vi "Power PID View.vi"(11 "Model in":refnum<class "Model.lvclass">) -> ()   [LabVIEW 2016, in "M1M3SupportEUI_Views.lvlib"]
uses:
  M1M3SupportEUI_Views.lvlib
  Model/Model.lvclass
  SALLV_m1m3/DataTypes/PIDData.ctl
  SALLV_m1m3/DataTypes/logevent_PIDInfo.ctl
  M1M3 Support Events/M1M3 Support Events.lvclass/M1M3 Support Events.ctl
  SALLV_m1m3/DataTypes/command_UpdatePID.ctl
  SALLV_m1m3/DataTypes/command_ResetPID.ctl
  SALLV_m1m3/DataTypes/command_TurnPowerOn.ctl
  M1M3 Support Events/M1M3 Support Events.lvclass
  SALLV_m1m3/SALLV_m1m3.lvlib
  EUI Events/EUI Events.lvclass
panel:
  out "Any":bool
  out "Power Warning Time Stamp":timestamp
  out "Power Status Time Stamp":timestamp
  out "AuxComDMismatch":bool
  out "MainComDMismatch":bool
  out "AuxComCMismatch":bool
  out "MainComCMismatch":bool
  out "AuxComBMismatch":bool
  out "MainComBMismatch":bool
  out "AuxComAMismatch":bool
  out "MainComAMismatch":bool
  out "AuxOutD":bool
  out "AuxOutC":bool
  out "AuxOutB":bool
  out "AuxOutA":bool
  out "AuxComD":bool
  out "AuxComC":bool
  out "AuxComB":bool
  out "AuxComA":bool
  out "MainOutD":bool
  out "MainOutC":bool
  out "MainOutB":bool
  out "MainOutA":bool
  out "MainComD":bool
  out "MainComC":bool
  out "MainComB":bool
  out "MainComA":bool
  in  "Aux All":bool
  in  "Aux D":bool
  in  "Aux C":bool
  in  "Aux B":bool
  in  "Aux A":bool
  in  "Main All":bool
  in  "Main D":bool
  in  "Main C":bool
  in  "Main B":bool
  in  "MainA":bool
  out "PID Event Time Stamp":timestamp
  in  "logevent_PIDInfo":T1={"Timestamp"=0.0, "Timestep[6]"=[0.0, 0.0, 0.0, 0.0, 0.0, 0.0], "P[6]"=[0.0, 0.0, 0.0, 0.0, 0.0, 0.0], "I[6]"=[0.0, 0.0, 0.0, 0.0, 0.0, 0.0], "D[6]"=[0.0, 0.0, 0.0, 0.0, 0.0, 0.0], "N[6]"=[0.0, 0.0, 0.0, 0.0, 0.0, 0.0], "CalculatedA[6]"=[0.0, 0.0, 0.0, 0.0, 0.0, 0.0], "CalculatedB[6]"=[0.0, 0.0, 0.0, 0.0, 0.0, 0.0], "CalculatedC[6]"=[0.0, 0.0, 0.0, 0.0, 0.0, 0.0], "CalculatedD[6]"=[0.0, 0.0, 0.0, 0.0, 0.0, 0.0], "CalculatedE[6]"=[0.0, 0.0, 0.0, 0.0, 0.0, 0.0], "priority"=0}
  in  "PID":enum16{"0", "1", "2", "3", "4", "5"}(ring)
  in  "N":dbl
  in  "D":dbl
  in  "I":dbl
  in  "P":dbl
  in  "Timestep":dbl
  in  "PID Data/Event Type":string(combo)
  out "6":string
  out "5":string
  out "4":string
  out "3":string
  out "2":string
  out "1":string
  in  "PIDData":T2={"Timestamp"=0.0, "Setpoint[6]"=[0.0, 0.0, 0.0, 0.0, 0.0, 0.0], "Measurement[6]"=[0.0, 0.0, 0.0, 0.0, 0.0, 0.0], "Error[6]"=[0.0, 0.0, 0.0, 0.0, 0.0, 0.0], "ErrorT1[6]"=[0.0, 0.0, 0.0, 0.0, 0.0, 0.0], "ErrorT2[6]"=[0.0, 0.0, 0.0, 0.0, 0.0, 0.0], "Control[6]"=[0.0, 0.0, 0.0, 0.0, 0.0, 0.0], "ControlT1[6]"=[0.0, 0.0, 0.0, 0.0, 0.0, 0.0], "ControlT2[6]"=[0.0, 0.0, 0.0, 0.0, 0.0, 0.0]}
  in  "Reset PID Button":bool
  in  "Update PID Button":bool
  out "Controls Power Network Current":string
  out "Light Power Network Current":string
  out "Power Network D Current":string
  out "Power Network C Current":string
  out "Power Network B Current":string
  out "Power Network A Current":string
  out "PID TelemetryTime Stamp":timestamp
  out "Power Time Stamp":timestamp
  # "Power"
  # "PID"
  # "Commands"
  # "Data"
  # "Commands"
  # "Main"
  # "Aux"
  # "PID"
  # "P"
  # "A"
  # "Timestep"
  # "I"
  # "B"
  # "C"
  # "D"
  # "D"
  # "N"
  # "ALL"
  # "Data & Events"
  # "Events"
  # "Status"
  # "Main"
  # "Auxiliary"
  # "Commanded"
  # "Commanded"
  # "Output"
  # "Output"
  # "A"
  # "3"
  # "1"
  # "2"
  # "B"
  # "C"
  # "6"
  # "4"
  # "5"
  # "D"
  # "Warnings - Mismatch"
  # "A"
  # "B"
  # "C"
  # "D"
  # "Main"
  # "Any -->"
  # "Auxiliary"
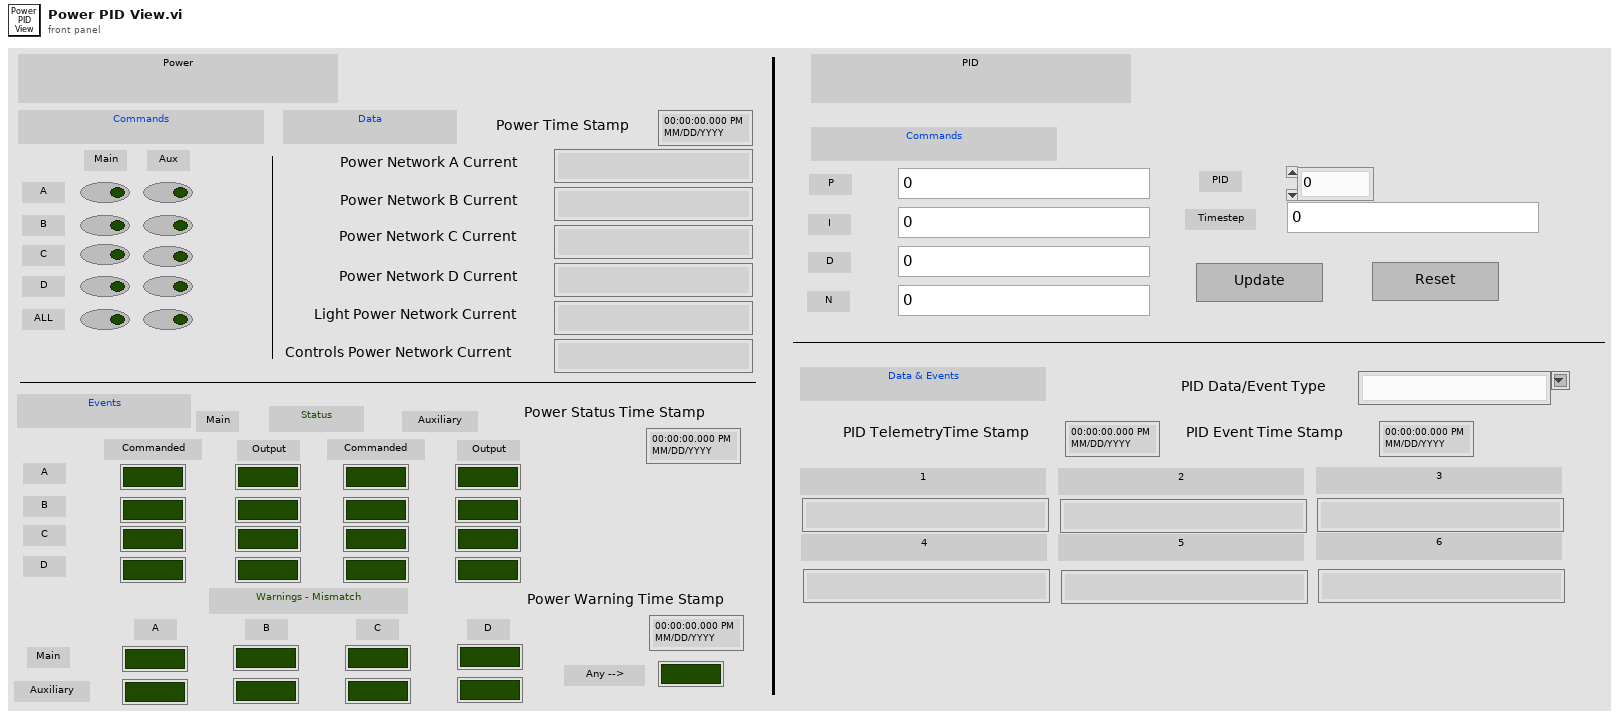
[diagram p1: front panel]
types:
  T1 = typedef "SALLV_m1m3.lvlib/logevent_PIDInfo.ctl" = cluster{"Timestamp":dbl, "Timestep[6]":dbl[], "P[6]":dbl[], "I[6]":dbl[], "D[6]":dbl[], "N[6]":dbl[], "CalculatedA[6]":dbl[], "CalculatedB[6]":dbl[], "CalculatedC[6]":dbl[], "CalculatedD[6]":dbl[], "CalculatedE[6]":dbl[], "priority":i32}
  T2 = typedef "SALLV_m1m3.lvlib/PIDData.ctl" = cluster{"Timestamp":dbl, "Setpoint[6]":dbl[], "Measurement[6]":dbl[], "Error[6]":dbl[], "ErrorT1[6]":dbl[], "ErrorT2[6]":dbl[], "Control[6]":dbl[], "ControlT1[6]":dbl[], "ControlT2[6]":dbl[]}
  T3 = typedef "M1M3SupportEUI_TypeDefs.lvlib/M1M3 Support Events.ctl" = cluster{"Inclinometer  Data":refnum<user-event>, "IMS Data":refnum<user-event>, "SAL Connected":refnum<user-event>, "Accelerometer Data":refnum<user-event>, "OuterLoop Data":refnum<user-event>, "ErrorCode Event":refnum<user-event>, "InterlockStatus Event":refnum<user-event>, "InterlockWarning Event":refnum<user-event>, "Gyro Data":refnum<user-event>, "HP Actuator Info Event":refnum<user-event>, " FA Info Event":refnum<user-event>, "HP Monitor Info Event":refnum<user-event>, "FA Data":refnum<user-event>, "HP Actuator data":refnum<user-event>, "HP Monitor data":refnum<user-event>, "Air Supply Status Event":refnum<user-event>, "Air Supply Warning Event":refnum<user-event>, "Power Data":refnum<user-event>, "PID Data":refnum<user-event>, "PID Info Event":refnum<user-event>, "Power Status Event":refnum<user-event>, "Power Supply Status Event":refnum<user-event>, "Power Warning Event":refnum<user-event>, "Summary State Event":refnum<user-event>, "Detailed State Event":refnum<user-event>, "FA Force Warning Event":refnum<user-event>, "FA Warning Event":refnum<user-event>, "FA State Event":refnum<user-event>, "Applied AberrationForces Event":refnum<user-event>, "Applied Acceleration Forcces Event":refnum<user-event>, "Applied Azimuth Forces Event":refnum<user-event>, "Applied Active Optic Forces Event":refnum<user-event>, "Applied Balance Forces Event":refnum<user-event>, "Applied Cylinder Forces Event":refnum<user-event>, "Applied Elevation Forces Event":refnum<user-event>, "Applied Forces Event":refnum<user-event>, "Applied Offset Forces Event":refnum<user-event>, "Applied Static Forces Event":refnum<user-event>, "Applied Thermal Forces Event":refnum<user-event>, "Applied Velocity Forces Event":refnum<user-event>, "Rejected Aberration Force Event":refnum<user-event>, "Rejected Acceleration Forces Event":refnum<user-event>, "Rejected Active Optic Forces Event":refnum<user-event>, "Rejected Azimuth Forces Event":refnum<user-event>, "Rejected Balance Forces Event":refnum<user-event>, "Rejected Cylinder Forces Event":refnum<user-event>, "Rejected Elevation Forces Event":refnum<user-event>, "Rejected Forces Event":refnum<user-event>, "Rejected Offset Forces Event":refnum<user-event>, "Rejected Static Forces Event":refnum<user-event>, "Rejected Thermal Forces Event":refnum<user-event>, "Rejected Velocity Forces Event":refnum<user-event>, "Command Rejection Event":refnum<user-event>, "Setting Verions Event":refnum<user-event>, "Settings Applied Event":refnum<user-event>, "HP Actuator State Event":refnum<user-event>, "HP Actuator Warning Event":refnum<user-event>, "HP Monitor State Event":refnum<user-event>, "HP Monitor Warning Event":refnum<user-event>, "Accelerometer Warning Event":refnum<user-event>, "Applied Settings Match Start Event":refnum<user-event>, "Cell Light Status Event ":refnum<user-event>, "Cell Light Warning Event":refnum<user-event>, "Displacement Sensor Warning Event":refnum<user-event>, "Force Setpoint Warning Event":refnum<user-event>, "Gyro Warning Event ":refnum<user-event>, "ILC Warning Event ":refnum<user-event>, "Inclinometer Sensor Warning Event ":refnum<user-event>}
  T4 = enum16{"", "DetailedState_DetailedStates_DisabledState", "DetailedState_DetailedStates_EnabledState", "DetailedState_DetailedStates_FaultState", "DetailedState_DetailedStates_OfflineState", "DetailedState_DetailedStates_StandbyState", "DetailedState_DetailedStates_ParkedState", "DetailedState_DetailedStates_RaisingState", "DetailedState_DetailedStates_ActiveState", "DetailedState_DetailedStates_LoweringState", "DetailedState_DetailedStates_EngineeringState", "DetailedState_DetailedStates_ParkedEngineeringState", "DetailedState_DetailedStates_RaisingEngineeringState", "DetailedState_DetailedStates_ActiveEngineeringState", "DetailedState_DetailedStates_LoweringEngineeringState", "DetailedState_DetailedStates_LoweringFaultState", "DetailedState_DetailedStates_ProfileHardpointCorrectionState"}
  T5 = typedef "SALLV_m1m3.lvlib/command_UpdatePID.ctl" = cluster{"PID":i16, "Timestep":dbl, "P":dbl, "I":dbl, "D":dbl, "N":dbl}
  T6 = typedef "SALLV_m1m3.lvlib/command_ResetPID.ctl" = cluster{"PID":i16}
  T7 = typedef "SALLV_m1m3.lvlib/command_TurnPowerOn.ctl" = cluster{"TurnPowerNetworkAOn":bool, "TurnPowerNetworkBOn":bool, "TurnPowerNetworkCOn":bool, "TurnPowerNetworkDOn":bool, "TurnAuxPowerNetworkAOn":bool, "TurnAuxPowerNetworkBOn":bool, "TurnAuxPowerNetworkCOn":bool, "TurnAuxPowerNetworkDOn":bool}
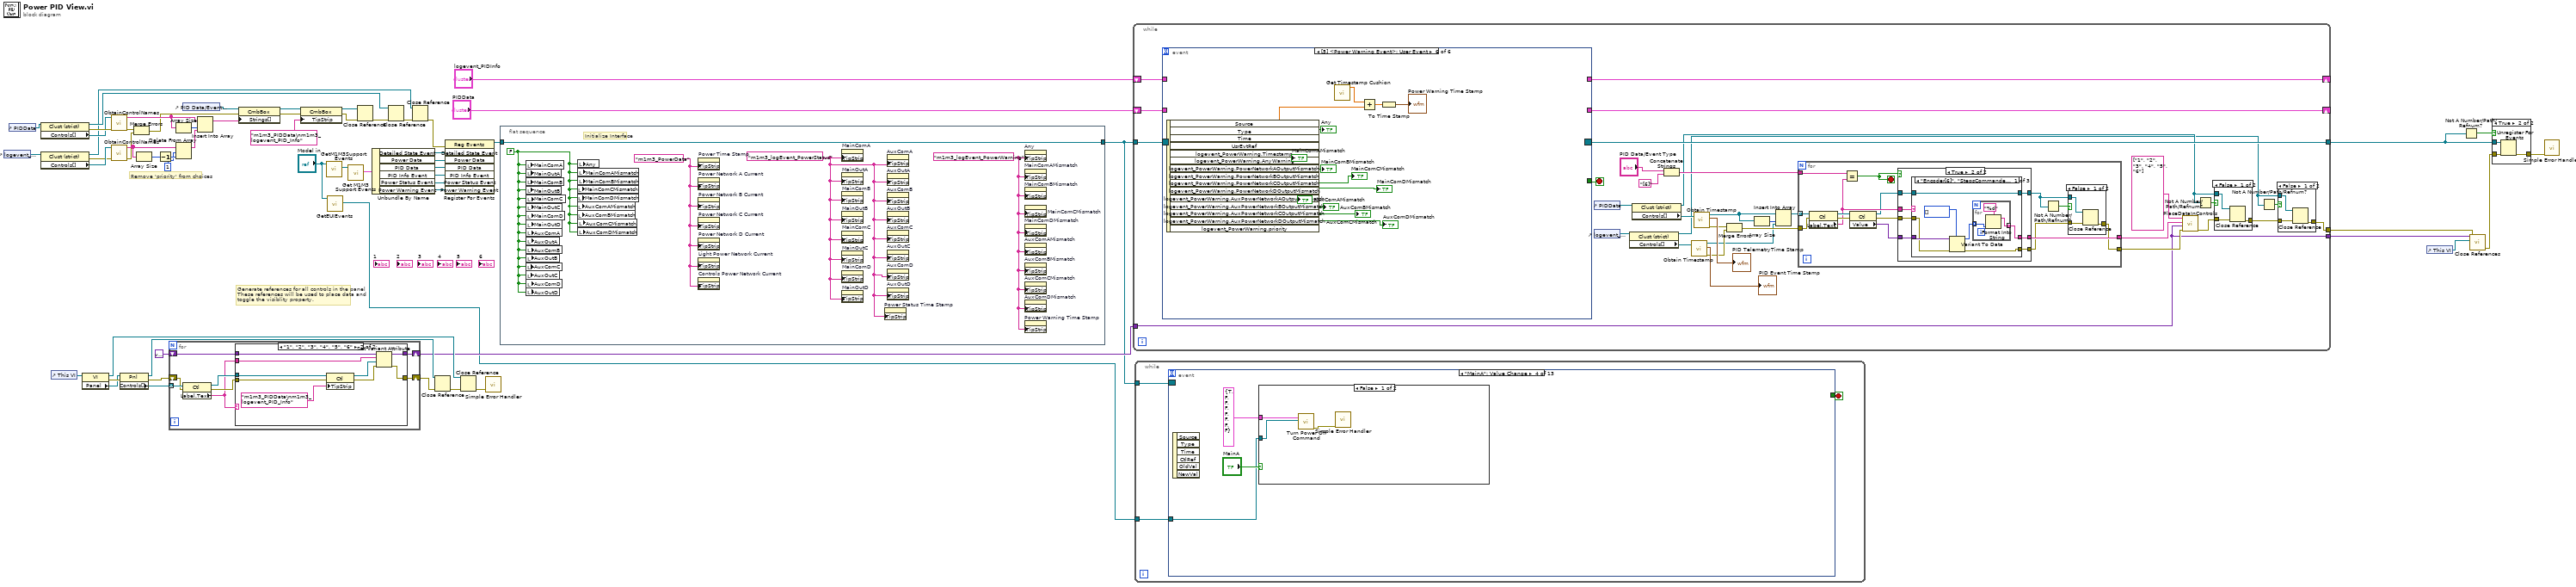
[diagram p0: block diagram]
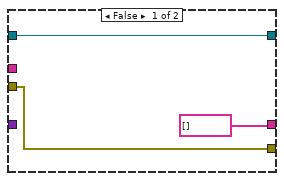
[diagram p4: hidden frame]
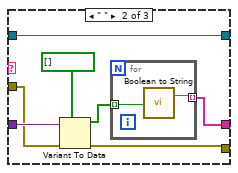
[diagram p5: hidden frame]
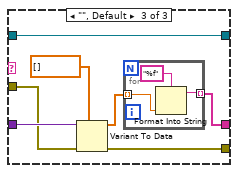
[diagram p6: hidden frame]
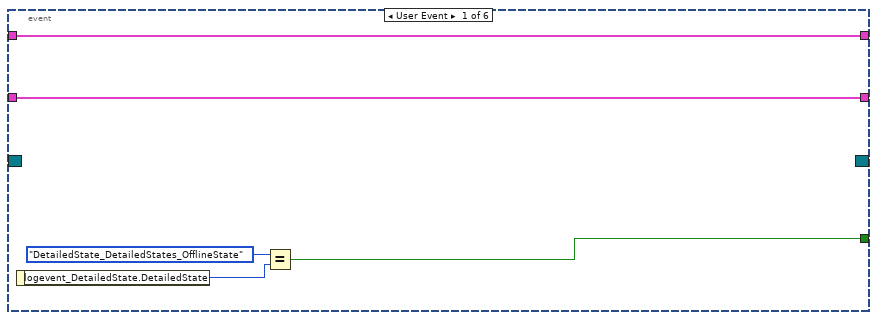
[diagram p7: hidden frame]
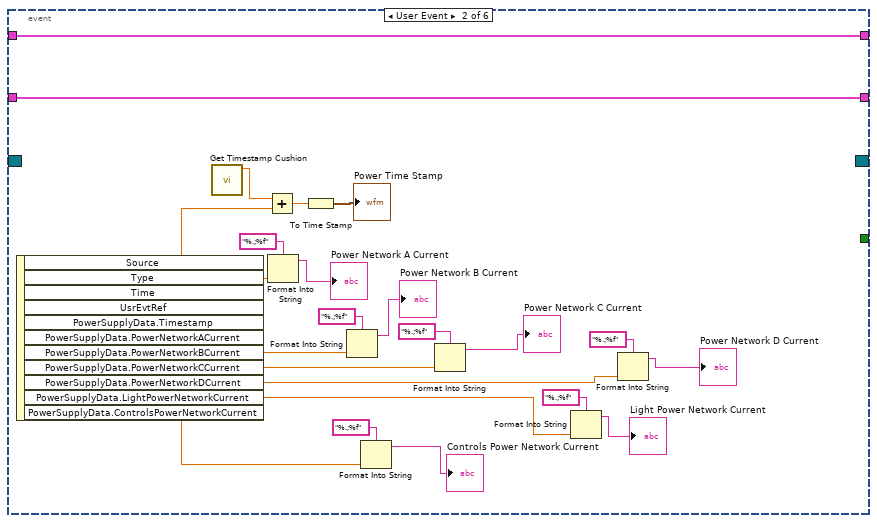
[diagram p8: hidden frame]
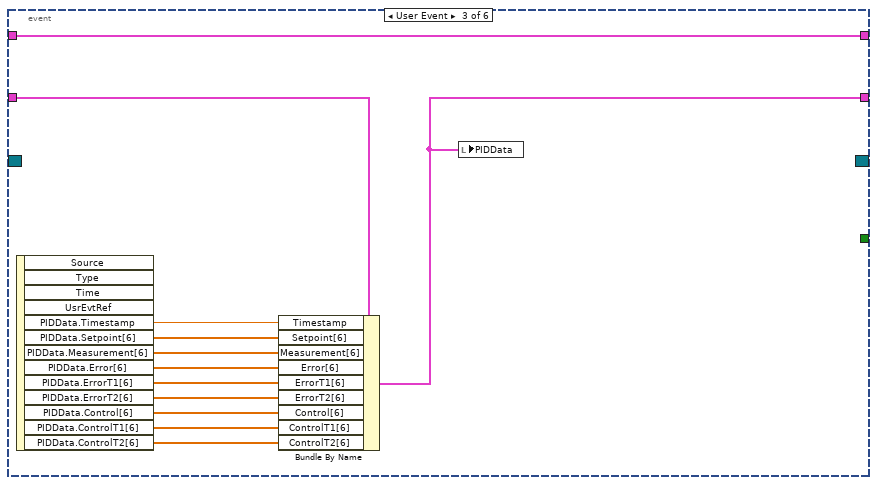
[diagram p9: hidden frame]
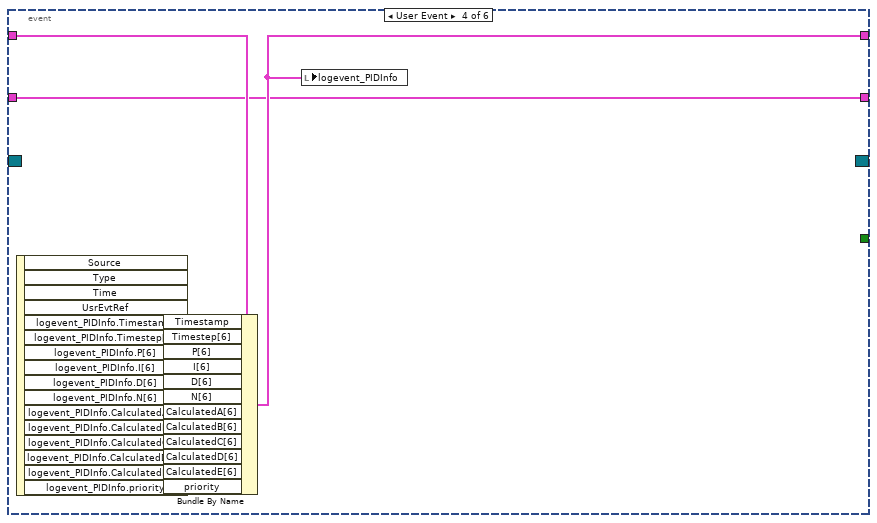
[diagram p10: hidden frame]
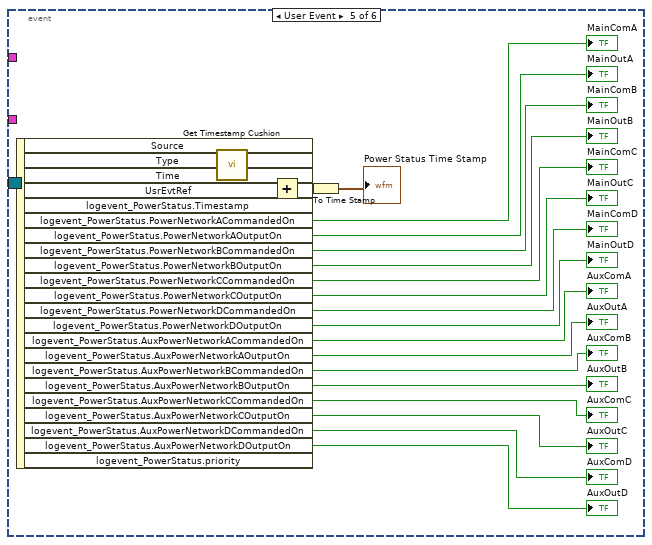
[diagram p11: hidden frame]
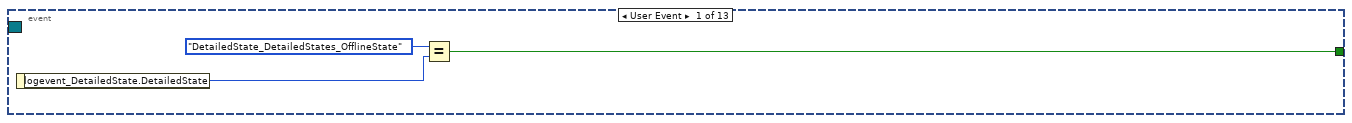
[diagram p14: hidden frame]
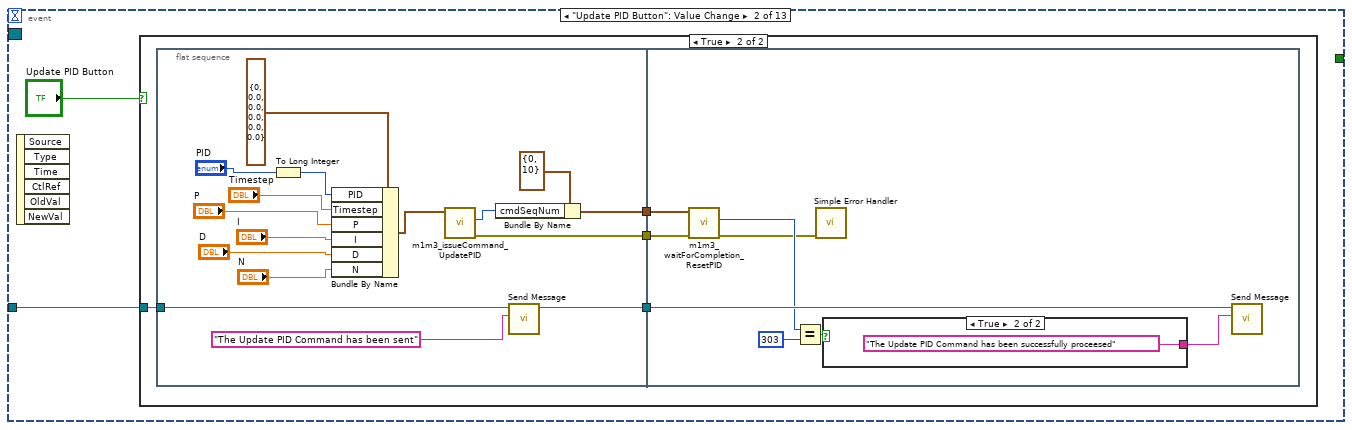
[diagram p15: hidden frame]
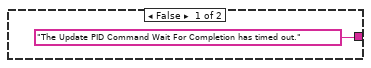
[diagram p17: hidden frame]
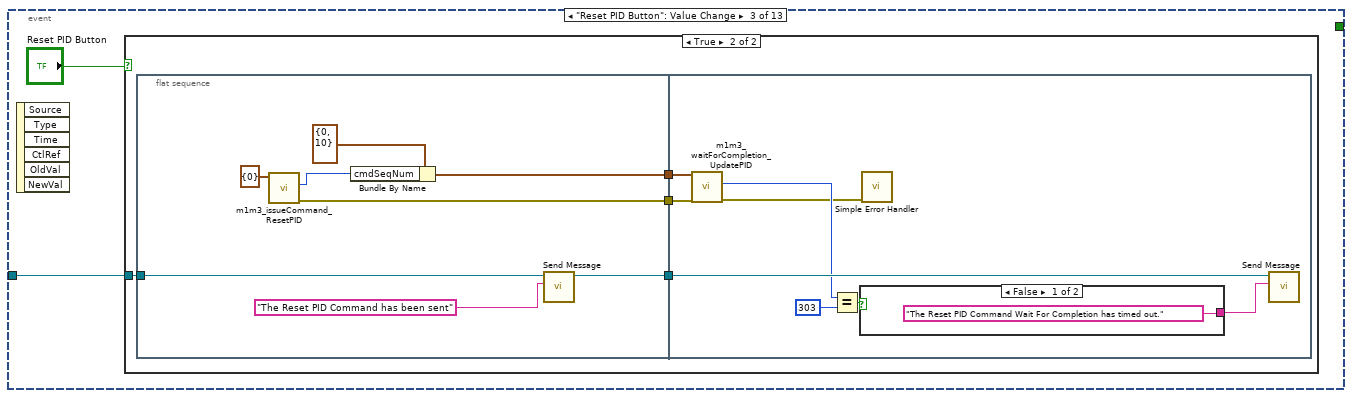
[diagram p18: hidden frame]
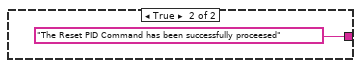
[diagram p20: hidden frame]
diagram:
  # "Remove 'priority' from choices"
  # "Generate references for all controls in the panel\nThese references will be used to place data and\ntoggle the visiblity property."
  n1 = control-ref of="logevent_PIDInfo"() -> (w25:refnum<vi>)
  n2 = control-ref of="PIDData"() -> (w54:refnum<vi>)
  n3 = property class="Clust (strict)"(reference=w54) -> (reference out=w46:refnum<vi>, error out=w55:errorcluster, "Controls[]"=w53:refnum<vi>[])  [unwired: 1 in]
  n4 = property class="Clust (strict)"(reference=w25) -> (reference out=w11:refnum<vi>, error out=w26:errorcluster, "Controls[]"=w27:refnum<vi>[])  [unwired: 1 in]
  n5 = control-ref of="This VI"() -> (w43:refnum<vi>)
  n6 = property class="VI"(reference=w43) -> (reference out=w34:refnum<vi>, error out=w42:errorcluster, "Panel"=w41:refnum<vi>)  [unwired: 1 in]
  n7 = call "ObtainControlNames.vi"("error in (no error)"=w55, "ControlRefnumArray"=w53) -> ("error out"=w21:errorcluster, "ControlNamesArray"=w22:string[])  [unwired: 8 in]
  n8 = call "ObtainControlNames.vi"("error in (no error)"=w26, "ControlRefnumArray"=w27) -> ("error out"=w19:errorcluster, "ControlNamesArray"=w17:string[])  [unwired: 8 in]
  n9 = property class="Pnl"(reference=w41, error in=w42) -> (reference out=w36:refnum<vi>, error out=w39:errorcluster, "Controls[]"=w40:refnum<vi>[])
  n10 = Merge Errors(w21, w19) -> (w20:errorcluster)
  n11 = Array Size(array=w17) -> (size(s)=w15:i32)
  n12 = Decrement(x=w15) -> (x-1=w16:i32)
  n13 = for {
    tunnel: w40 -> [w69] mode=indexing
    shift-right: [w65] -> w37
    shift-left: w39 -> [w67]
    shift-right: [w63] -> w33
    shift-left: variant -> [w64]
    n14 = property class="Ctl"(reference=w69, error in=w67) -> (reference out=w68:refnum<vi>, error out=w66:errorcluster, "Label.Text"=w62:string)
    n15 = case shown="\"1\", \"2\", \"3\", \"4\", \"5\", \"6\"" w62 {
      tunnel: w62 -> [_ w78]
      tunnel: w68 -> [_ w75]
      tunnel: w66 -> [w70 w74]
      tunnel: [w70 w77] -> w65
      tunnel: w64 -> [w71 w80]
      tunnel: [w71 w79] -> w63
      frame "", Default {
      }
      frame "1", "2", "3", "4", "5", "6" {
        n16 = property class="Ctl"(reference=w75, error in=w74, "TipStrip"="m1m3_PIDData\nm1m3_logevent_PID_Info") -> (reference out=w73:refnum<vi>, error out=w72:errorcluster)
        n17 = Set Variant Attribute(Variant=w80, name=w78, value=w73, error in=w72) -> (Variant out=w79:variant, error out=w77:errorcluster)  [unwired: 1 out]
      }
    }
  }
  n18 = Delete From Array(array=w17, length=1, index=w16) -> (array with subset deleted=w18:string[])  [unwired: 1 out]
  n19 = Array Size(array=w22) -> (size(s)=w24:i32)
  n20 = control-ref of="PID Data/Event Type"() -> (w49:refnum<vi>)
  n21 = Insert Into Array(array=w22, index=w24, new element=w18) -> (w23:string[])
  n22 = property class="CmbBox"(reference=w49, error in=w20, "Strings[]"=w23) -> (reference out=w50:refnum<vi>, error out=w51:errorcluster)
  n23 = property class="CmbBox"(reference=w50, error in=w51, "TipStrip"="m1m3_PIDData\nm1m3_logevent_PID_Info") -> (reference out=w48:refnum<vi>, error out=w47:errorcluster)
  n24 = call "GetM1M3SupportEvents.vi"("Model in"="Model in") -> ("M1M3 Support Events out"=w57:refnum<class "M1M3 Support Events.lvclass">)  [unwired: 8 in, 2 out]
  n25 = call "GetEUIEvents.vi"("Model in"="Model in") -> ("EUI Events out"=w1:refnum<class "EUI Events.lvclass">)  [unwired: 8 in, 2 out]
  n26 = call "Get M1M3 Support Events.vi"("M1M3 Support Events in"=w57) -> ("M1M3 Support Events"=w58:T3)  [unwired: 9 in, 1 out]
  n27 = Close Reference(reference=w48, error in (no error)=w47) -> (error out=w45:errorcluster)
  n28 = Unbundle By Name(w58) -> ("Detailed State Event"=w59:refnum<user-event>, "Power Data"=w60:refnum<user-event>, "PID Data"=w61:refnum<user-event>, "PID Info Event"=w29:refnum<user-event>, "Power Status Event"=w10:refnum<user-event>, "Power Warning Event"=w9:refnum<user-event>)
  n29 = Close Reference(reference=w46, error in (no error)=w45) -> (error out=w13:errorcluster)
  n30 = Close Reference(reference=w11, error in (no error)=w13) -> (error out=w12:errorcluster)
  n31 = Close Reference(reference=w36, error in (no error)=w37) -> (error out=w38:errorcluster)
  n32 = register-events(error in=w12, w59, w60, w61, w29, w10, w9) -> (reference out=w8:refnum<event-registration>)  [unwired: 1 in, 1 out]
  n33 = Close Reference(reference=w34, error in (no error)=w38) -> (error out=w35:errorcluster)
  n34 = call <vilib>:"Simple Error Handler.vi"("error in (no error)"=w35) -> ()  [unwired: 4 in, 5 out]
  n35 = flat-sequence {
    tunnel: [w85] -> w7
    tunnel: w8 -> [w85]
    frame #0 {
      w81 = "m1m3_logEvent_PowerWarning" ("Tip Strip")
      w82 = "m1m3_logEvent_PowerStatus" ("Tip Strip")
      w83 = "m1m3_PowerData" ("Tip Strip")
      w84 = FALSE
      # "Initialize Interface"
      n36 = local write "MainComA"(w84) -> ()
      n37 = local write "MainOutA"(w84) -> ()
      n38 = local write "MainComB"(w84) -> ()
      n39 = local write "MainOutB"(w84) -> ()
      n40 = local write "AuxComC"(w84) -> ()
      n41 = local write "AuxOutC"(w84) -> ()
      n42 = local write "MainComC"(w84) -> ()
      n43 = local write "MainOutC"(w84) -> ()
      n44 = local write "MainComD"(w84) -> ()
      n45 = local write "MainOutD"(w84) -> ()
      n46 = local write "AuxComA"(w84) -> ()
      n47 = local write "AuxOutA"(w84) -> ()
      n48 = local write "AuxComB"(w84) -> ()
      n49 = local write "AuxOutB"(w84) -> ()
      n50 = local write "AuxComD"(w84) -> ()
      n51 = local write "AuxOutD"(w84) -> ()
      n52 = local write "MainComCMismatch"(w84) -> ()
      n53 = local write "MainComDMismatch"(w84) -> ()
      n54 = local write "AuxComAMismatch"(w84) -> ()
      n55 = local write "AuxComBMismatch"(w84) -> ()
      n56 = local write "Any"(w84) -> ()
      n57 = local write "MainComAMismatch"(w84) -> ()
      n58 = local write "MainComBMismatch"(w84) -> ()
      n59 = local write "AuxComCMismatch"(w84) -> ()
      n60 = local write "AuxComDMismatch"(w84) -> ()
      n61 = property on="Power Time Stamp" class="AbsTime (strict)"("TipStrip"=w83) -> ()  [unwired: 2 in, 2 out]
      n62 = property on="Power Network A Current" class="Str"("TipStrip"=w83) -> ()  [unwired: 2 in, 2 out]
      n63 = property on="Power Network B Current" class="Str"("TipStrip"=w83) -> ()  [unwired: 2 in, 2 out]
      n64 = property on="Power Network C Current" class="Str"("TipStrip"=w83) -> ()  [unwired: 2 in, 2 out]
      n65 = property on="Power Network D Current" class="Str"("TipStrip"=w83) -> ()  [unwired: 2 in, 2 out]
      n66 = property on="Light Power Network Current" class="Str"("TipStrip"=w83) -> ()  [unwired: 2 in, 2 out]
      n67 = property on="Controls Power Network Current" class="Str"("TipStrip"=w83) -> ()  [unwired: 2 in, 2 out]
      n68 = property on="MainComA" class="Bool (strict)"("TipStrip"=w82) -> ()  [unwired: 2 in, 2 out]
      n69 = property on="MainOutA" class="Bool (strict)"("TipStrip"=w82) -> ()  [unwired: 2 in, 2 out]
      n70 = property on="MainComB" class="Bool (strict)"("TipStrip"=w82) -> ()  [unwired: 2 in, 2 out]
      n71 = property on="MainOutB" class="Bool (strict)"("TipStrip"=w82) -> ()  [unwired: 2 in, 2 out]
      n72 = property on="MainComC" class="Bool (strict)"("TipStrip"=w82) -> ()  [unwired: 2 in, 2 out]
      n73 = property on="MainOutC" class="Bool (strict)"("TipStrip"=w82) -> ()  [unwired: 2 in, 2 out]
      n74 = property on="MainComD" class="Bool (strict)"("TipStrip"=w82) -> ()  [unwired: 2 in, 2 out]
      n75 = property on="MainOutD" class="Bool (strict)"("TipStrip"=w82) -> ()  [unwired: 2 in, 2 out]
      n76 = property on="Power Status Time Stamp" class="AbsTime (strict)"("TipStrip"=w82) -> ()  [unwired: 2 in, 2 out]
      n77 = property on="AuxComA" class="Bool (strict)"("TipStrip"=w82) -> ()  [unwired: 2 in, 2 out]
      n78 = property on="AuxOutA" class="Bool (strict)"("TipStrip"=w82) -> ()  [unwired: 2 in, 2 out]
      n79 = property on="AuxComB" class="Bool (strict)"("TipStrip"=w82) -> ()  [unwired: 2 in, 2 out]
      n80 = property on="AuxOutB" class="Bool (strict)"("TipStrip"=w82) -> ()  [unwired: 2 in, 2 out]
      n81 = property on="AuxComC" class="Bool (strict)"("TipStrip"=w82) -> ()  [unwired: 2 in, 2 out]
      n82 = property on="AuxOutC" class="Bool (strict)"("TipStrip"=w82) -> ()  [unwired: 2 in, 2 out]
      n83 = property on="AuxComD" class="Bool (strict)"("TipStrip"=w82) -> ()  [unwired: 2 in, 2 out]
      n84 = property on="AuxOutD" class="Bool (strict)"("TipStrip"=w82) -> ()  [unwired: 2 in, 2 out]
      n85 = property on="Any" class="Bool (strict)"("TipStrip"=w81) -> ()  [unwired: 2 in, 2 out]
      n86 = property on="MainComAMismatch" class="Bool (strict)"("TipStrip"=w81) -> ()  [unwired: 2 in, 2 out]
      n87 = property on="MainComBMismatch" class="Bool (strict)"("TipStrip"=w81) -> ()  [unwired: 2 in, 2 out]
      n88 = property on="MainComCMismatch" class="Bool (strict)"("TipStrip"=w81) -> ()  [unwired: 2 in, 2 out]
      n89 = property on="MainComDMismatch" class="Bool (strict)"("TipStrip"=w81) -> ()  [unwired: 2 in, 2 out]
      n90 = property on="AuxComAMismatch" class="Bool (strict)"("TipStrip"=w81) -> ()  [unwired: 2 in, 2 out]
      n91 = property on="AuxComBMismatch" class="Bool (strict)"("TipStrip"=w81) -> ()  [unwired: 2 in, 2 out]
      n92 = property on="AuxComCMismatch" class="Bool (strict)"("TipStrip"=w81) -> ()  [unwired: 2 in, 2 out]
      n93 = property on="AuxComDMismatch" class="Bool (strict)"("TipStrip"=w81) -> ()  [unwired: 2 in, 2 out]
      n94 = property on="Power Warning Time Stamp" class="AbsTime (strict)"("TipStrip"=w81) -> ()  [unwired: 2 in, 2 out]
    }
  }
  n95 = while {
    tunnel: w7 -> [w119]
    shift-right: [w116] -> _
    shift-left: "PIDData" -> [w117]
    tunnel: [w115] -> w5
    tunnel: w33 -> [w105]
    tunnel: [w87] -> w31
    tunnel: [w105] -> w30
    shift-right: [w103] -> _
    shift-left: "logevent_PIDInfo" -> [w104]
    stop <- w118 stop-if-true
    n96 = event shown="[5] <Power Warning Event>: User Event" {
      selector: w119 -> [_ _ _ _ _ _]
      dyn-events: [_ _ _ _ _ _] -> w115
      timeout: _ -> [_ _ _ _ _ _]
      tunnel: [w182 _ _ _ _ _] -> w118
      tunnel: w117 -> [w181 w184 w218 w220 _ _]
      tunnel: [w181 w184 w209 w220 _ _] -> w116
      tunnel: w104 -> [w180 w183 w207 w233 _ _]
      tunnel: [w180 w183 w207 w221 _ _] -> w103
      event User Event {
        n97 = event-data() -> ("logevent_DetailedState.DetailedState"=w179:T4)  [unwired: 1 in]
        n98 = Equal?(x=T4."DetailedState_DetailedStates_OfflineState", y=w179) -> (x = y?=w182:bool)
      }
      event User Event {
        n99 = event-data() -> ("PowerSupplyData.Timestamp"=w204:dbl, "PowerSupplyData.PowerNetworkACurrent"=w202:sgl, "PowerSupplyData.PowerNetworkBCurrent"=w196:sgl, "PowerSupplyData.PowerNetworkCCurrent"=w194:sgl, "PowerSupplyData.PowerNetworkDCurrent"=w192:sgl, "PowerSupplyData.LightPowerNetworkCurrent"=w189:sgl, "PowerSupplyData.ControlsPowerNetworkCurrent"=w186:sgl)  [unwired: 1 in, 4 out]
        n100 = call "Get Timestamp Cushion.vi"() -> ("TimestampCushion"=w206:dbl)  [unwired: 11 in]
        n101 = Add(x=w206, y=w204) -> (x+y=w205:dbl)
        n102 = Format Into String(format string="%.;%f", w202) -> (resulting string=→"Power Network A Current":string)  [unwired: 2 in, 1 out]
        n103 = To Time Stamp(1:w205) -> (0:→"Power Time Stamp":timestamp)
        n104 = Format Into String(format string="%.;%f", w196) -> (resulting string=→"Power Network B Current":string)  [unwired: 2 in, 1 out]
        n105 = Format Into String(format string="%.;%f", w186) -> (resulting string=→"Controls Power Network Current":string)  [unwired: 2 in, 1 out]
        n106 = Format Into String(format string="%.;%f", w194) -> (resulting string=→"Power Network C Current":string)  [unwired: 2 in, 1 out]
        n107 = Format Into String(format string="%.;%f", w189) -> (resulting string=→"Light Power Network Current":string)  [unwired: 2 in, 1 out]
        n108 = Format Into String(format string="%.;%f", w192) -> (resulting string=→"Power Network D Current":string)  [unwired: 2 in, 1 out]
      }
      event User Event {
        n109 = event-data() -> ("PIDData.Timestamp"=w208:dbl, "PIDData.Setpoint[6]"=w217:dbl[], "PIDData.Measurement[6]"=w216:dbl[], "PIDData.Error[6]"=w215:dbl[], "PIDData.ErrorT1[6]"=w214:dbl[], "PIDData.ErrorT2[6]"=w213:dbl[], "PIDData.Control[6]"=w212:dbl[], "PIDData.ControlT1[6]"=w211:dbl[], "PIDData.ControlT2[6]"=w210:dbl[])  [unwired: 1 in, 4 out]
        n110 = Bundle By Name(cluster=w218, "Timestamp"=w208, "Setpoint[6]"=w217, "Measurement[6]"=w216, "Error[6]"=w215, "ErrorT1[6]"=w214, "ErrorT2[6]"=w213, "Control[6]"=w212, "ControlT1[6]"=w211, "ControlT2[6]"=w210) -> (w209:T2)
        n111 = local write "PIDData"(w209) -> ()
      }
      event User Event {
        n112 = event-data() -> ("logevent_PIDInfo.Timestamp"=w232:dbl, "logevent_PIDInfo.Timestep[6]"=w231:dbl[], "logevent_PIDInfo.P[6]"=w230:dbl[], "logevent_PIDInfo.I[6]"=w229:dbl[], "logevent_PIDInfo.D[6]"=w228:dbl[], "logevent_PIDInfo.N[6]"=w227:dbl[], "logevent_PIDInfo.CalculatedA[6]"=w226:dbl[], "logevent_PIDInfo.CalculatedB[6]"=w225:dbl[], "logevent_PIDInfo.CalculatedC[6]"=w224:dbl[], "logevent_PIDInfo.CalculatedD[6]"=w223:dbl[], "logevent_PIDInfo.CalculatedE[6]"=w222:dbl[], "logevent_PIDInfo.priority"=w219:i32)  [unwired: 1 in, 4 out]
        n113 = Bundle By Name(cluster=w233, "Timestamp"=w232, "Timestep[6]"=w231, "P[6]"=w230, "I[6]"=w229, "D[6]"=w228, "N[6]"=w227, "CalculatedA[6]"=w226, "CalculatedB[6]"=w225, "CalculatedC[6]"=w224, "CalculatedD[6]"=w223, "CalculatedE[6]"=w222, "priority"=w219) -> (w221:T1)
        n114 = local write "logevent_PIDInfo"(w221) -> ()
      }
      event User Event {
        n115 = event-data() -> ("logevent_PowerStatus.Timestamp"=w235:dbl, "logevent_PowerStatus.PowerNetworkACommandedOn"=→"MainComA":bool, "logevent_PowerStatus.PowerNetworkAOutputOn"=→"MainOutA":bool, "logevent_PowerStatus.PowerNetworkBCommandedOn"=→"MainComB":bool, "logevent_PowerStatus.PowerNetworkBOutputOn"=→"MainOutB":bool, "logevent_PowerStatus.PowerNetworkCCommandedOn"=→"MainComC":bool, "logevent_PowerStatus.PowerNetworkCOutputOn"=→"MainOutC":bool, "logevent_PowerStatus.PowerNetworkDCommandedOn"=→"MainComD":bool, "logevent_PowerStatus.PowerNetworkDOutputOn"=→"MainOutD":bool, "logevent_PowerStatus.AuxPowerNetworkACommandedOn"=→"AuxComA":bool, "logevent_PowerStatus.AuxPowerNetworkAOutputOn"=→"AuxOutA":bool, "logevent_PowerStatus.AuxPowerNetworkBCommandedOn"=→"AuxComB":bool, "logevent_PowerStatus.AuxPowerNetworkBOutputOn"=→"AuxOutB":bool, "logevent_PowerStatus.AuxPowerNetworkCCommandedOn"=→"AuxComC":bool, "logevent_PowerStatus.AuxPowerNetworkCOutputOn"=→"AuxOutC":bool, "logevent_PowerStatus.AuxPowerNetworkDCommandedOn"=→"AuxComD":bool, "logevent_PowerStatus.AuxPowerNetworkDOutputOn"=→"AuxOutD":bool)  [unwired: 1 in, 5 out]
        n116 = call "Get Timestamp Cushion.vi"() -> ("TimestampCushion"=w236:dbl)  [unwired: 11 in]
        n117 = Add(x=w236, y=w235) -> (x+y=w237:dbl)
        n118 = To Time Stamp(1:w237) -> (0:→"Power Status Time Stamp":timestamp)
      }
      event User Event {
        n119 = event-data() -> ("logevent_PowerWarning.Timestamp"=w255:dbl, "logevent_PowerWarning.AnyWarning"=→"Any":bool, "logevent_PowerWarning.PowerNetworkAOutputMismatch"=→"MainComAMismatch":bool, "logevent_PowerWarning.PowerNetworkBOutputMismatch"=→"MainComBMismatch":bool, "logevent_PowerWarning.PowerNetworkCOutputMismatch"=→"MainComCMismatch":bool, "logevent_PowerWarning.PowerNetworkDOutputMismatch"=→"MainComDMismatch":bool, "logevent_PowerWarning.AuxPowerNetworkAOutputMismatch"=→"AuxComAMismatch":bool, "logevent_PowerWarning.AuxPowerNetworkBOutputMismatch"=→"AuxComBMismatch":bool, "logevent_PowerWarning.AuxPowerNetworkCOutputMismatch"=→"AuxComCMismatch":bool, "logevent_PowerWarning.AuxPowerNetworkDOutputMismatch"=→"AuxComDMismatch":bool)  [unwired: 1 in, 5 out]
        n120 = call "Get Timestamp Cushion.vi"() -> ("TimestampCushion"=w256:dbl)  [unwired: 11 in]
        n121 = Add(x=w256, y=w255) -> (x+y=w257:dbl)
        n122 = To Time Stamp(1:w257) -> (0:→"Power Warning Time Stamp":timestamp)
      }
    }
    n123 = control-ref of="PIDData"() -> (w113:refnum<vi>)
    n124 = control-ref of="logevent_PIDInfo"() -> (w101:refnum<vi>)
    n125 = property class="Clust (strict)"(reference=w101) -> (reference out=w86:refnum<vi>, "Controls[]"=w102:refnum<vi>[])  [unwired: 1 in, 1 out]
    n126 = property class="Clust (strict)"(reference=w113) -> (reference out=w90:refnum<vi>, "Controls[]"=w114:refnum<vi>[])  [unwired: 1 in, 1 out]
    n127 = Concatenate Strings("PID Data/Event Type", "[6]" ("string")) -> (w109:string)
    n128 = call "Obtain Timestamp.vi"("ControlRefnumArray"=w102) -> ("error out"=w98:errorcluster, "Time Stamp"=→"PID Event Time Stamp":timestamp, "Array"=w93:refnum<vi>[])  [unwired: 8 in]
    n129 = call "Obtain Timestamp.vi"("ControlRefnumArray"=w114) -> ("error out"=w99:errorcluster, "Time Stamp"=→"PID TelemetryTime Stamp":timestamp, "Array"=w95:refnum<vi>[])  [unwired: 8 in]
    n130 = Merge Errors(w99, w98) -> (w97:errorcluster)
    n131 = Array Size(array=w95) -> (size(s)=w96:i32)
    n132 = Insert Into Array(array=w95, index=w96, new element=w93) -> (w94:refnum<vi>[])
    n133 = for {
      tunnel: w109 -> [w128]
      tunnel: w94 -> [w133] mode=indexing
      tunnel: [w120] -> w106
      tunnel: [w126] -> w107
      tunnel: w97 -> [w124]
      stop <- w130 stop-if-true
      n134 = property class="Ctl"(reference=w133, error in=w124) -> (reference out=w131:refnum<vi>, error out=w132:errorcluster, "Label.Text"=w127:string)
      n135 = Equal?(x=w128, y=w127) -> (x = y?=w130:bool)
      n136 = property class="Ctl"(reference=w131, error in=w132) -> (reference out=w125:refnum<vi>, error out=w129:errorcluster, "Value"=w134:variant)
      n137 = case shown="True" w130 {
        tunnel: w134 -> [_ w148]
        tunnel: w127 -> [_ w147]
        tunnel: w129 -> [w141 w146]
        tunnel: [w141 w145] -> w121
        tunnel: [string[] [] w144] -> w126
        tunnel: w125 -> [w139 w143]
        tunnel: [w139 w142] -> w122
        frame False {
        }
        frame True {
          n138 = case shown="\"Encoder[6]\", \"StepsCommanded[6]\", \"StepsQueued[6]\"" w147 {
            tunnel: w148 -> [w154 w164 w174]
            tunnel: [w150 w160 w169] -> w144
            tunnel: w146 -> [w153 w163 w172]
            tunnel: [w152 w162 w171] -> w145
            tunnel: w143 -> [w149 w159 w168]
            tunnel: [w149 w159 w168] -> w142
            frame "Encoder[6]", "StepsCommanded[6]", "StepsQueued[6]" {
              n139 = Variant To Data(error in=w153, type=i32[] [], Variant=w154) -> (data=w151:i32[], error out=w152:errorcluster)
              n140 = for {
                tunnel: w151 -> [w158] mode=indexing
                tunnel: [w157] -> w150 mode=indexing
                n141 = Format Into String(format string="%d", w158) -> (resulting string=w157:string)  [unwired: 2 in, 1 out]
              }
            }
            frame " " {
              n142 = Variant To Data(error in=w163, type=bool[] [], Variant=w164) -> (data=w161:bool[], error out=w162:errorcluster)
              n143 = for {
                tunnel: w161 -> [w167] mode=indexing
                tunnel: [w166] -> w160 mode=indexing
                n144 = call "Boolean to String.vi"("BooleanValue"=w167) -> ("StringForm"=w166:string)  [unwired: 1 out]
              }
            }
            frame "", Default {
              n145 = Variant To Data(error in=w172, type=dbl[] [], Variant=w174) -> (data=w170:dbl[], error out=w171:errorcluster)
              n146 = for {
                tunnel: w170 -> [w177] mode=indexing
                tunnel: [w176] -> w169 mode=indexing
                n147 = Format Into String(format string="%f", w177) -> (resulting string=w176:string)  [unwired: 2 in, 1 out]
              }
            }
          }
        }
      }
      n148 = Not A Number/Path/Refnum?(number/path/refnum=w122) -> (NaN/Path/Refnum?=w123:bool)
      n149 = case shown="False" w123 {
        tunnel: w121 -> [w137 w138]
        tunnel: [w136 w138] -> w120
        tunnel: w122 -> [w135 _]
        frame False {
          n150 = Close Reference(reference=w135, error in (no error)=w137) -> (error out=w136:errorcluster)
        }
        frame True {
        }
      }
    }
    n151 = call "PlaceDataInControls.vi"("error in (no error)"=w106, "Variant"=w105, "DataArray"=w107, "ControlNamesArray"=string[] ["1", "2", "3", "4", "5", "6"]) -> ("error out"=w91:errorcluster)  [unwired: 7 in]
    n152 = Not A Number/Path/Refnum?(number/path/refnum=w90) -> (NaN/Path/Refnum?=w92:bool)
    n153 = case shown="False" w92 {
      tunnel: w91 -> [w269 w270]
      tunnel: [w268 w270] -> w88
      tunnel: w90 -> [w267 _]
      frame False {
        n154 = Close Reference(reference=w267, error in (no error)=w269) -> (error out=w268:errorcluster)
      }
      frame True {
      }
    }
    n155 = Not A Number/Path/Refnum?(number/path/refnum=w86) -> (NaN/Path/Refnum?=w89:bool)
    n156 = case shown="False" w89 {
      tunnel: w88 -> [w273 w274]
      tunnel: [w272 w274] -> w87
      tunnel: w86 -> [w271 _]
      frame False {
        n157 = Close Reference(reference=w271, error in (no error)=w273) -> (error out=w272:errorcluster)
      }
      frame True {
      }
    }
  }
  n158 = while {
    tunnel: w7 -> [w277]
    tunnel: w1 -> [w275]
    stop <- w276 stop-if-true
    n159 = event shown="[3] \"MainA\": Value Change" {
      selector: w277 -> [_ _ _ _ _ _ _ _ _ _ _ _ _]
      dyn-events: _ -> [_ _ _ _ _ _ _ _ _ _ _ _ _]
      timeout: _ -> [_ _ _ _ _ _ _ _ _ _ _ _ _]
      tunnel: [w280 _ _ _ _ _ _ _ _ _ _ _ _] -> w276
      tunnel: w275 -> [_ w281 w313 w337 w346 w355 w364 w373 w384 w393 w402 w411 w420]
      event User Event {
        n160 = event-data() -> ("logevent_DetailedState.DetailedState"=w279:T4)  [unwired: 1 in]
        n161 = Equal?(x=T4."DetailedState_DetailedStates_OfflineState", y=w279) -> (x = y?=w280:bool)
      }
      event "Update PID Button": Value Change {
        n162 = event-data() -> ()  [unwired: 1 in, 6 out]
        n163 = case shown="True" "Update PID Button" {
          tunnel: w281 -> [_ w286]
          frame False {
          }
          frame True {
            n164 = flat-sequence {
              tunnel: w286 -> [w290]
              tunnel: [w289] -> w285
              tunnel: [w288] -> w284
              tunnel: [w287] -> w283
              tunnel: w285 -> [w307]
              tunnel: w284 -> [w306]
              tunnel: w283 -> [w305]
              frame #0 {
                n165 = To Long Integer(number="PID") -> (32bit integer=w293:i32)
                n166 = Bundle By Name(cluster=T5 {"PID"=0, "Timestep"=0.0, "P"=0.0, "I"=0.0, "D"=0.0, "N"=0.0} ("command_UpdatePID_Ctl"), "PID"=w293, "Timestep"="Timestep", "P"="P", "I"="I", "D"="D", "N"="N") -> (w301:T5)
                n167 = call "m1m3_issueCommand_UpdatePID.vi"("command_UpdatePID_Ctl"=w301) -> ("error out"=w288:errorcluster, "function return"=w299:i32)  [unwired: 8 in, 1 out]
                n168 = Bundle By Name(cluster=cluster{"cmdSeqNum":i32, "timeout":u32} {"cmdSeqNum"=0, "timeout"=10} ("waitComplete_Ctl"), "cmdSeqNum"=w299) -> (w287:cluster{"cmdSeqNum":i32, "timeout":u32})
                n169 = call "Send Message.vi"("Message"="The Update PID Command has been sent", "EUI Events in"=w290) -> ("EUI Events out"=w289:refnum<class "EUI Events.lvclass">)  [unwired: 8 in, 1 out]
              }
              frame #1 {
                n170 = call "m1m3_waitForCompletion_ResetPID.vi"("error in (no error)"=w306, "waitComplete_Ctl"=w305) -> ("error out"=w303:errorcluster, "function return"=w304:i32)  [unwired: 7 in, 1 out]
                n171 = Equal?(x=w304, y=303) -> (x = y?=w309:bool)
                n172 = call <vilib>:"Simple Error Handler.vi"("error in (no error)"=w303) -> ()  [unwired: 4 in, 5 out]
                n173 = case shown="True" w309 {
                  tunnel: ["The Update PID Command Wait For Completion has timed out." ("Message") "The Update PID Command has been successfully proceesed" ("Message")] -> w310
                  frame False {
                  }
                  frame True {
                  }
                }
                n174 = call "Send Message.vi"("Message"=w310, "EUI Events in"=w307) -> ()  [unwired: 8 in, 2 out]
              }
            }
          }
        }
      }
      event "Reset PID Button": Value Change {
        n175 = event-data() -> ()  [unwired: 1 in, 6 out]
        n176 = case shown="True" "Reset PID Button" {
          tunnel: w313 -> [_ w318]
          frame False {
          }
          frame True {
            n177 = flat-sequence {
              tunnel: w318 -> [w322]
              tunnel: [w321] -> w317
              tunnel: [w320] -> w316
              tunnel: [w319] -> w315
              tunnel: w317 -> [w331]
              tunnel: w316 -> [w330]
              tunnel: w315 -> [w329]
              frame #0 {
                n178 = call "m1m3_issueCommand_ResetPID.vi"("command_ResetPID_Ctl"=T6 {"PID"=0}) -> ("error out"=w320:errorcluster, "function return"=w324:i32)  [unwired: 8 in, 1 out]
                n179 = Bundle By Name(cluster=cluster{"cmdSeqNum":i32, "timeout":u32} {"cmdSeqNum"=0, "timeout"=10} ("waitComplete_Ctl"), "cmdSeqNum"=w324) -> (w319:cluster{"cmdSeqNum":i32, "timeout":u32})
                n180 = call "Send Message.vi"("Message"="The Reset PID Command has been sent", "EUI Events in"=w322) -> ("EUI Events out"=w321:refnum<class "EUI Events.lvclass">)  [unwired: 8 in, 1 out]
              }
              frame #1 {
                n181 = call "m1m3_waitForCompletion_UpdatePID.vi"("error in (no error)"=w330, "waitComplete_Ctl"=w329) -> ("error out"=w327:errorcluster, "function return"=w328:i32)  [unwired: 7 in, 1 out]
                n182 = Equal?(x=w328, y=303) -> (x = y?=w333:bool)
                n183 = case shown="False" w333 {
                  tunnel: ["The Reset PID Command Wait For Completion has timed out." ("Message") "The Reset PID Command has been successfully proceesed" ("Message")] -> w334
                  frame False {
                  }
                  frame True {
                  }
                }
                n184 = call <vilib>:"Simple Error Handler.vi"("error in (no error)"=w327) -> ()  [unwired: 4 in, 5 out]
                n185 = call "Send Message.vi"("Message"=w334, "EUI Events in"=w331) -> ()  [unwired: 8 in, 2 out]
              }
            }
          }
        }
      }
      event "MainA": Value Change {
        n186 = event-data() -> ()  [unwired: 1 in, 6 out]
        n187 = case shown="False" "MainA" {
          tunnel: T7 {"TurnPowerNetworkAOn"=TRUE, "TurnPowerNetworkBOn"=FALSE, "TurnPowerNetworkCOn"=FALSE, "TurnPowerNetworkDOn"=FALSE, "TurnAuxPowerNetworkAOn"=FALSE, "TurnAuxPowerNetworkBOn"=FALSE, "TurnAuxPowerNetworkCOn"=FALSE, "TurnAuxPowerNetworkDOn"=FALSE} ("command_TurnPowerOn_Ctl") -> [w342 w345]
          tunnel: w337 -> [w341 w344]
          frame False {
            n188 = call "Turn Power Off Command.vi"("EUI Events.lvclass"=w341, "command_TurnPowerOff"=w342) -> ("error out"=w340:errorcluster)  [unwired: 9 in]
            n189 = call <vilib>:"Simple Error Handler.vi"("error in (no error)"=w340) -> ()  [unwired: 4 in, 5 out]
          }
          frame True {
            n190 = call "Turn Power On Command.vi"("EUI Events.lvclass"=w344, "command_TurnPowerOn"=w345) -> ("error out"=w343:errorcluster)  [unwired: 9 in]
            n191 = call <vilib>:"Simple Error Handler.vi"("error in (no error)"=w343) -> ()  [unwired: 4 in, 5 out]
          }
        }
      }
      event "Main B": Value Change {
        n192 = event-data() -> ()  [unwired: 1 in, 6 out]
        n193 = case shown="False" "Main B" {
          tunnel: T7 {"TurnPowerNetworkAOn"=FALSE, "TurnPowerNetworkBOn"=TRUE, "TurnPowerNetworkCOn"=FALSE, "TurnPowerNetworkDOn"=FALSE, "TurnAuxPowerNetworkAOn"=FALSE, "TurnAuxPowerNetworkBOn"=FALSE, "TurnAuxPowerNetworkCOn"=FALSE, "TurnAuxPowerNetworkDOn"=FALSE} ("command_TurnPowerOn_Ctl") -> [w351 w354]
          tunnel: w346 -> [w350 w353]
          frame False {
            n194 = call "Turn Power Off Command.vi"("EUI Events.lvclass"=w350, "command_TurnPowerOff"=w351) -> ("error out"=w349:errorcluster)  [unwired: 9 in]
            n195 = call <vilib>:"Simple Error Handler.vi"("error in (no error)"=w349) -> ()  [unwired: 4 in, 5 out]
          }
          frame True {
            n196 = call "Turn Power On Command.vi"("EUI Events.lvclass"=w353, "command_TurnPowerOn"=w354) -> ("error out"=w352:errorcluster)  [unwired: 9 in]
            n197 = call <vilib>:"Simple Error Handler.vi"("error in (no error)"=w352) -> ()  [unwired: 4 in, 5 out]
          }
        }
      }
      event "Main C": Value Change {
        n198 = event-data() -> ()  [unwired: 1 in, 6 out]
        n199 = case shown="False" "Main C" {
          tunnel: T7 {"TurnPowerNetworkAOn"=FALSE, "TurnPowerNetworkBOn"=FALSE, "TurnPowerNetworkCOn"=TRUE, "TurnPowerNetworkDOn"=FALSE, "TurnAuxPowerNetworkAOn"=FALSE, "TurnAuxPowerNetworkBOn"=FALSE, "TurnAuxPowerNetworkCOn"=FALSE, "TurnAuxPowerNetworkDOn"=FALSE} ("command_TurnPowerOn_Ctl") -> [w360 w363]
          tunnel: w355 -> [w359 w362]
          frame False {
            n200 = call "Turn Power Off Command.vi"("EUI Events.lvclass"=w359, "command_TurnPowerOff"=w360) -> ("error out"=w358:errorcluster)  [unwired: 9 in]
            n201 = call <vilib>:"Simple Error Handler.vi"("error in (no error)"=w358) -> ()  [unwired: 4 in, 5 out]
          }
          frame True {
            n202 = call "Turn Power On Command.vi"("EUI Events.lvclass"=w362, "command_TurnPowerOn"=w363) -> ("error out"=w361:errorcluster)  [unwired: 9 in]
            n203 = call <vilib>:"Simple Error Handler.vi"("error in (no error)"=w361) -> ()  [unwired: 4 in, 5 out]
          }
        }
      }
      event "Main D": Value Change {
        n204 = event-data() -> ()  [unwired: 1 in, 6 out]
        n205 = case shown="True" "Main D" {
          tunnel: T7 {"TurnPowerNetworkAOn"=FALSE, "TurnPowerNetworkBOn"=FALSE, "TurnPowerNetworkCOn"=FALSE, "TurnPowerNetworkDOn"=TRUE, "TurnAuxPowerNetworkAOn"=FALSE, "TurnAuxPowerNetworkBOn"=FALSE, "TurnAuxPowerNetworkCOn"=FALSE, "TurnAuxPowerNetworkDOn"=FALSE} ("command_TurnPowerOn_Ctl") -> [w369 w372]
          tunnel: w364 -> [w368 w371]
          frame False {
            n206 = call "Turn Power Off Command.vi"("EUI Events.lvclass"=w368, "command_TurnPowerOff"=w369) -> ("error out"=w367:errorcluster)  [unwired: 9 in]
            n207 = call <vilib>:"Simple Error Handler.vi"("error in (no error)"=w367) -> ()  [unwired: 4 in, 5 out]
          }
          frame True {
            n208 = call "Turn Power On Command.vi"("EUI Events.lvclass"=w371, "command_TurnPowerOn"=w372) -> ("error out"=w370:errorcluster)  [unwired: 9 in]
            n209 = call <vilib>:"Simple Error Handler.vi"("error in (no error)"=w370) -> ()  [unwired: 4 in, 5 out]
          }
        }
      }
      event "Main All": Value Change {
        n210 = event-data() -> ()  [unwired: 1 in, 6 out]
        n211 = case shown="False" "Main All" {
          tunnel: T7 {"TurnPowerNetworkAOn"=TRUE, "TurnPowerNetworkBOn"=TRUE, "TurnPowerNetworkCOn"=TRUE, "TurnPowerNetworkDOn"=TRUE, "TurnAuxPowerNetworkAOn"=FALSE, "TurnAuxPowerNetworkBOn"=FALSE, "TurnAuxPowerNetworkCOn"=FALSE, "TurnAuxPowerNetworkDOn"=FALSE} ("command_TurnPowerOn_Ctl") -> [w379 w383]
          tunnel: w373 -> [w377 w381]
          frame False {
            w378 = FALSE
            n212 = call "Turn Power Off Command.vi"("EUI Events.lvclass"=w377, "command_TurnPowerOff"=w379) -> ("error out"=w376:errorcluster)  [unwired: 9 in]
            n213 = call <vilib>:"Simple Error Handler.vi"("error in (no error)"=w376) -> ()  [unwired: 4 in, 5 out]
            n214 = local write "MainA"(w378) -> ()
            n215 = local write "Main B"(w378) -> ()
            n216 = local write "Main C"(w378) -> ()
            n217 = local write "Main D"(w378) -> ()
          }
          frame True {
            w382 = TRUE
            n218 = call "Turn Power On Command.vi"("EUI Events.lvclass"=w381, "command_TurnPowerOn"=w383) -> ("error out"=w380:errorcluster)  [unwired: 9 in]
            n219 = call <vilib>:"Simple Error Handler.vi"("error in (no error)"=w380) -> ()  [unwired: 4 in, 5 out]
            n220 = local write "MainA"(w382) -> ()
            n221 = local write "Main B"(w382) -> ()
            n222 = local write "Main C"(w382) -> ()
            n223 = local write "Main D"(w382) -> ()
          }
        }
      }
      event "Aux A": Value Change {
        n224 = event-data() -> ()  [unwired: 1 in, 6 out]
        n225 = case shown="True" "Aux A" {
          tunnel: T7 {"TurnPowerNetworkAOn"=FALSE, "TurnPowerNetworkBOn"=FALSE, "TurnPowerNetworkCOn"=FALSE, "TurnPowerNetworkDOn"=FALSE, "TurnAuxPowerNetworkAOn"=TRUE, "TurnAuxPowerNetworkBOn"=FALSE, "TurnAuxPowerNetworkCOn"=FALSE, "TurnAuxPowerNetworkDOn"=FALSE} ("command_TurnPowerOn_Ctl") -> [w389 w392]
          tunnel: w384 -> [w388 w391]
          frame False {
            n226 = call "Turn Power Off Command.vi"("EUI Events.lvclass"=w388, "command_TurnPowerOff"=w389) -> ("error out"=w387:errorcluster)  [unwired: 9 in]
            n227 = call <vilib>:"Simple Error Handler.vi"("error in (no error)"=w387) -> ()  [unwired: 4 in, 5 out]
          }
          frame True {
            n228 = call "Turn Power On Command.vi"("EUI Events.lvclass"=w391, "command_TurnPowerOn"=w392) -> ("error out"=w390:errorcluster)  [unwired: 9 in]
            n229 = call <vilib>:"Simple Error Handler.vi"("error in (no error)"=w390) -> ()  [unwired: 4 in, 5 out]
          }
        }
      }
      event "Aux B": Value Change {
        n230 = event-data() -> ()  [unwired: 1 in, 6 out]
        n231 = case shown="True" "Aux B" {
          tunnel: T7 {"TurnPowerNetworkAOn"=FALSE, "TurnPowerNetworkBOn"=FALSE, "TurnPowerNetworkCOn"=FALSE, "TurnPowerNetworkDOn"=FALSE, "TurnAuxPowerNetworkAOn"=FALSE, "TurnAuxPowerNetworkBOn"=TRUE, "TurnAuxPowerNetworkCOn"=FALSE, "TurnAuxPowerNetworkDOn"=FALSE} ("command_TurnPowerOn_Ctl") -> [w398 w401]
          tunnel: w393 -> [w397 w400]
          frame False {
            n232 = call "Turn Power Off Command.vi"("EUI Events.lvclass"=w397, "command_TurnPowerOff"=w398) -> ("error out"=w396:errorcluster)  [unwired: 9 in]
            n233 = call <vilib>:"Simple Error Handler.vi"("error in (no error)"=w396) -> ()  [unwired: 4 in, 5 out]
          }
          frame True {
            n234 = call "Turn Power On Command.vi"("EUI Events.lvclass"=w400, "command_TurnPowerOn"=w401) -> ("error out"=w399:errorcluster)  [unwired: 9 in]
            n235 = call <vilib>:"Simple Error Handler.vi"("error in (no error)"=w399) -> ()  [unwired: 4 in, 5 out]
          }
        }
      }
      event "Aux C": Value Change {
        n236 = event-data() -> ()  [unwired: 1 in, 6 out]
        n237 = case shown="True" "Aux C" {
          tunnel: T7 {"TurnPowerNetworkAOn"=FALSE, "TurnPowerNetworkBOn"=FALSE, "TurnPowerNetworkCOn"=FALSE, "TurnPowerNetworkDOn"=FALSE, "TurnAuxPowerNetworkAOn"=FALSE, "TurnAuxPowerNetworkBOn"=FALSE, "TurnAuxPowerNetworkCOn"=TRUE, "TurnAuxPowerNetworkDOn"=FALSE} ("command_TurnPowerOn_Ctl") -> [w407 w410]
          tunnel: w402 -> [w406 w408]
          frame False {
            n238 = call "Turn Power Off Command.vi"("EUI Events.lvclass"=w406, "command_TurnPowerOff"=w407) -> ("error out"=w405:errorcluster)  [unwired: 9 in]
            n239 = call <vilib>:"Simple Error Handler.vi"("error in (no error)"=w405) -> ()  [unwired: 4 in, 5 out]
          }
          frame True {
            n240 = call "Turn Power On Command.vi"("EUI Events.lvclass"=w408, "command_TurnPowerOn"=w410) -> ("error out"=w409:errorcluster)  [unwired: 9 in]
            n241 = call <vilib>:"Simple Error Handler.vi"("error in (no error)"=w409) -> ()  [unwired: 4 in, 5 out]
          }
        }
      }
      event "Aux D": Value Change {
        n242 = event-data() -> ()  [unwired: 1 in, 6 out]
        n243 = case shown="True" "Aux D" {
          tunnel: T7 {"TurnPowerNetworkAOn"=FALSE, "TurnPowerNetworkBOn"=FALSE, "TurnPowerNetworkCOn"=FALSE, "TurnPowerNetworkDOn"=FALSE, "TurnAuxPowerNetworkAOn"=FALSE, "TurnAuxPowerNetworkBOn"=FALSE, "TurnAuxPowerNetworkCOn"=FALSE, "TurnAuxPowerNetworkDOn"=TRUE} ("command_TurnPowerOn_Ctl") -> [w416 w419]
          tunnel: w411 -> [w415 w417]
          frame False {
            n244 = call "Turn Power Off Command.vi"("EUI Events.lvclass"=w415, "command_TurnPowerOff"=w416) -> ("error out"=w414:errorcluster)  [unwired: 9 in]
            n245 = call <vilib>:"Simple Error Handler.vi"("error in (no error)"=w414) -> ()  [unwired: 4 in, 5 out]
          }
          frame True {
            n246 = call "Turn Power On Command.vi"("EUI Events.lvclass"=w417, "command_TurnPowerOn"=w419) -> ("error out"=w418:errorcluster)  [unwired: 9 in]
            n247 = call <vilib>:"Simple Error Handler.vi"("error in (no error)"=w418) -> ()  [unwired: 4 in, 5 out]
          }
        }
      }
      event "Aux All": Value Change {
        n248 = event-data() -> ()  [unwired: 1 in, 6 out]
        n249 = case shown="True" "Aux All" {
          tunnel: T7 {"TurnPowerNetworkAOn"=FALSE, "TurnPowerNetworkBOn"=FALSE, "TurnPowerNetworkCOn"=FALSE, "TurnPowerNetworkDOn"=FALSE, "TurnAuxPowerNetworkAOn"=TRUE, "TurnAuxPowerNetworkBOn"=TRUE, "TurnAuxPowerNetworkCOn"=TRUE, "TurnAuxPowerNetworkDOn"=TRUE} ("command_TurnPowerOn_Ctl") -> [w426 w430]
          tunnel: w420 -> [w423 w428]
          frame False {
            w425 = FALSE
            n250 = call "Turn Power Off Command.vi"("EUI Events.lvclass"=w423, "command_TurnPowerOff"=w426) -> ("error out"=w424:errorcluster)  [unwired: 9 in]
            n251 = call <vilib>:"Simple Error Handler.vi"("error in (no error)"=w424) -> ()  [unwired: 4 in, 5 out]
            n252 = local write "Aux C"(w425) -> ()
            n253 = local write "Aux B"(w425) -> ()
            n254 = local write "Aux A"(w425) -> ()
            n255 = local write "Aux D"(w425) -> ()
          }
          frame True {
            w429 = TRUE
            n256 = call "Turn Power On Command.vi"("EUI Events.lvclass"=w428, "command_TurnPowerOn"=w430) -> ("error out"=w427:errorcluster)  [unwired: 9 in]
            n257 = call <vilib>:"Simple Error Handler.vi"("error in (no error)"=w427) -> ()  [unwired: 4 in, 5 out]
            n258 = local write "Aux B"(w429) -> ()
            n259 = local write "Aux C"(w429) -> ()
            n260 = local write "Aux D"(w429) -> ()
            n261 = local write "Aux A"(w429) -> ()
          }
        }
      }
    }
  }
  n262 = control-ref of="This VI"() -> (w32:refnum<vi>)
  n263 = Not A Number/Path/Refnum?(number/path/refnum=w5) -> (NaN/Path/Refnum?=w6:bool)
  n264 = call "Close References.vi"("error in (no error)"=w31, "VI Refnum"=w32, "Variant"=w30) -> ("error out"=w4:errorcluster)  [unwired: 8 in]
  n265 = case shown="True" w6 {
    tunnel: w5 -> [_ w434]
    tunnel: w4 -> [w431 w433]
    tunnel: [w431 w432] -> w3
    frame False {
    }
    frame True {
      n266 = Unregister For Events(event registration refnum=w434, error in=w433) -> (error out=w432:errorcluster)
    }
  }
  n267 = call <vilib>:"Simple Error Handler.vi"("error in (no error)"=w3) -> ()  [unwired: 4 in, 5 out]
